vi "NTCP Link Status DAO.vi"(8 "error in (no error)":errorcluster, 9 "NTCP Link In":bool, 11 "DAO Actions":T1=enum."Get") -> (0 "error out":errorcluster, 1 "NTCP Link Out":bool)   [LabVIEW 2013]
uses:
  Data Access Objects/Metadata/DAO Actions.ctl
  IPC Messages/Offset Message Type.ctl
  Offsets/GlobalOrLocal.ctl
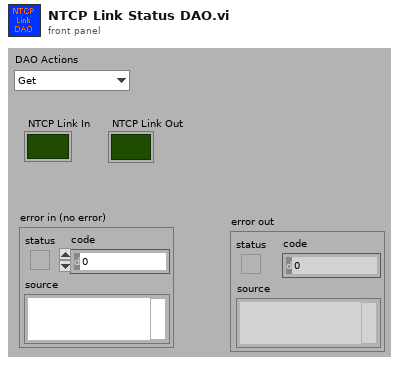
[diagram p1: front panel]
types:
  T1 = typedef "DAO Actions.ctl" = enum16{"Init", "Get", "Set"}
  T2 = typedef "Offset Message Type.ctl" = cluster{"Cartesian Type":T3, "Force Tag":string}
  T3 = typedef "GlobalOrLocal.ctl" = bool
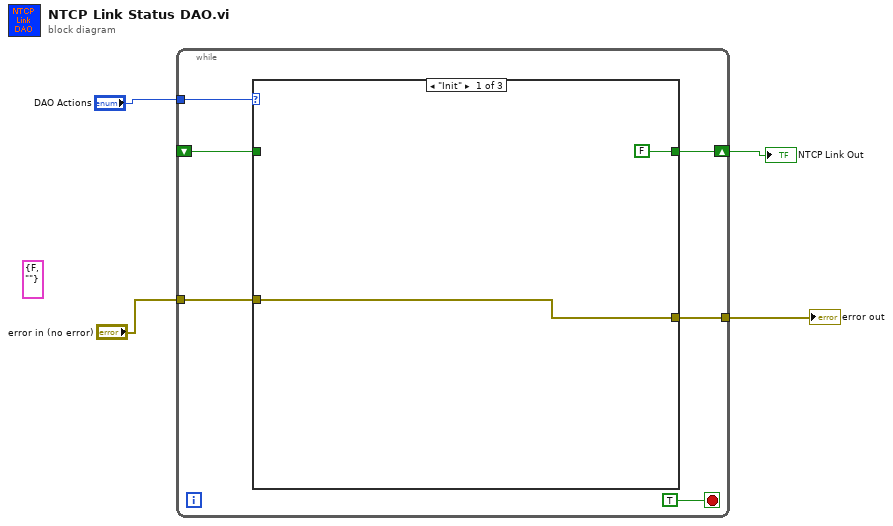
[diagram p0: block diagram]
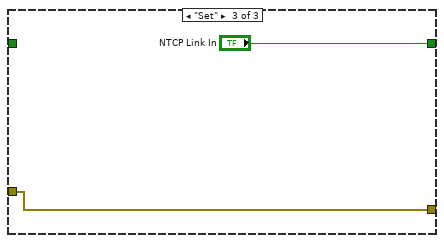
[diagram p3: hidden frame]
diagram:
  (unwired) T2 {"Cartesian Type"=FALSE, "Force Tag"=""} ("Offset In")
  n1 = while {
    tunnel: "DAO Actions" -> [w10]
    tunnel: "error in (no error)" -> [w9]
    tunnel: [w8] -> w2
    shift-right: [w7] -> w1
    shift-left: _ -> [w6]
    stop <- TRUE stop-if-true
    n2 = case shown="\"Init\"" w10 {
      tunnel: w9 -> [w11 w13 w15]
      tunnel: [w11 w13 w15] -> w8
      tunnel: [FALSE w14 "NTCP Link In"] -> w7
      tunnel: w6 -> [_ w14 _]
      frame "Init" {
      }
      frame "Get" {
      }
      frame "Set" {
      }
    }
  }
  "NTCP Link Out" <- w1
  "error out" <- w2
